vi "ServerPolicy.vi"(3 "xml content":string="<?xml version=\"1.0\" encoding=\"utf-8\"?><opcua_server><name>Faraday Cup Control System</name><port>4845</port><policy>none</policy><serverCertification></serverCertification><trustedClientCertifications>  <certification></certification></trustedClientCertifications><structure>    <folder name=\"System\">        <item name=\"Server URL\" ,access=\"read/write\" datatype=\"string\" initialValue=\"\" description=\"Server URL.\"></item>    </folder>    <folder name=\"Motion\">        <folder name=\"Contorl\">            <item name=\"Power Enable\" access=\"read/write\" datatype=\"boolean\" initialValue=\"FALSE\" description=\"Enable the motion power.\"></item>            <item name=\"Start Move\" access=\"read/write\" datatype=\"boolean\" initialValue=\"FALSE\" description=\"Start to move.\"></item>            <item name=\"Stop Move\" access=\"read/write\" datatype=\"boolean\" initialValue=\"FALSE\" description=\"Stop the movement.\"></item>            <item name=\"Find Home\" access=\"read/write\" datatype=\"boolean\" initialValue=\"FALSE\" description=\"Start to find home.\"></item>        </folder>        <folder name=\"Status\">            <item name=\"FWD Limit\" access=\"read\" datatype=\"boolean\" initialValue=\"FALSE\" description=\"Show the status of fwd limit.\"></item>            <item name=\"REV Limit\" access=\"read\" datatype=\"boolean\" initialValue=\"FALSE\" description=\"Show the status of rev limit.\"></item>            <item name=\"STO\" access=\"read\" datatype=\"boolean\" initialValue=\"FALSE\" description=\"Show the status of STO.\"></item>            <item name=\"Move Complete\" access=\"read\" datatype=\"boolean\" initialValue=\"FALSE\" description=\"Show the status of movement.\"></item>            <item name=\"Find Home Complete\" access=\"read\" datatype=\"boolean\" initialValue=\"FALSE\" description=\"show the status of finding home.\"></item>            <item name=\"E Ruler\" access=\"read\" datatype=\"double\" initialValue=\"0\" description=\"Show the Eruler position.\"></item>        </folder>        <folder name=\"Last Error\">            <item name=\"acknowledge\" access=\"read/write\" datatype=\"boolean\" initialValue=\"FALSE\" description=\"Acknowledge last error.\"></item>            <item name=\"code\" access=\"read\" datatype=\"int32\" initialValue=\"0\" description=\"Show the code of last error.\"></item>            <item name=\"info\" access=\"read\" datatype=\"int32\" initialValue=\"0\" description=\"Show the info of last error.\"></item>        </folder>    </folder>    <folder name=\"DAQ\">        <item name=\"Measurement Range\" access=\"read/write\" datatype=\"int16\" initialValue=\"100\" description=\"Measurement range.\"></item>        <item name=\"Intensity\" access=\"read\" datatype=\"double\" initialValue=\"100\" description=\"Intensity Value.\"></item>        <item name=\"Save file?\" access=\"read/write\" datatype=\"boolean\" initialValue=\"FALSE\" description=\"Enable saving file.\"></item>        <item name=\"File Path\" access=\"read/write\" datatype=\"string\" initialValue=\"\" description=\"Local path of saved file.\"></item>    </folder></structure></opcua_server>") -> (0 "security policy":T1, 1 "xml content(dup)":string)   [LabVIEW 2013, in "OPCUA XML.lvlib"]
uses:
  OPCUA XML.lvlib
panel:
  out "result string":string
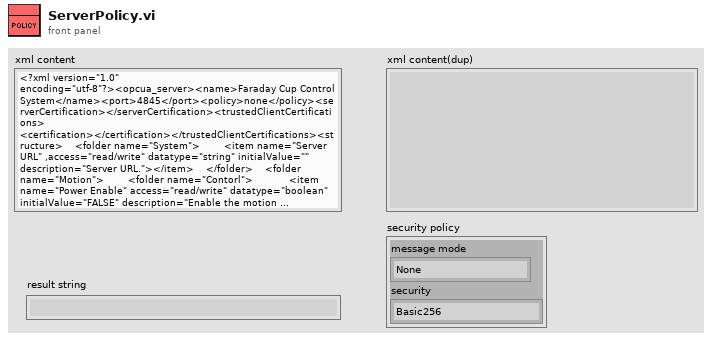
[diagram p1: front panel]
types:
  T1 = cluster{"message mode":enum16{"None", "Sign", "Sign and Encrypt"}, "security":enum16{"Basic256", "Basic128Rsa15"}}
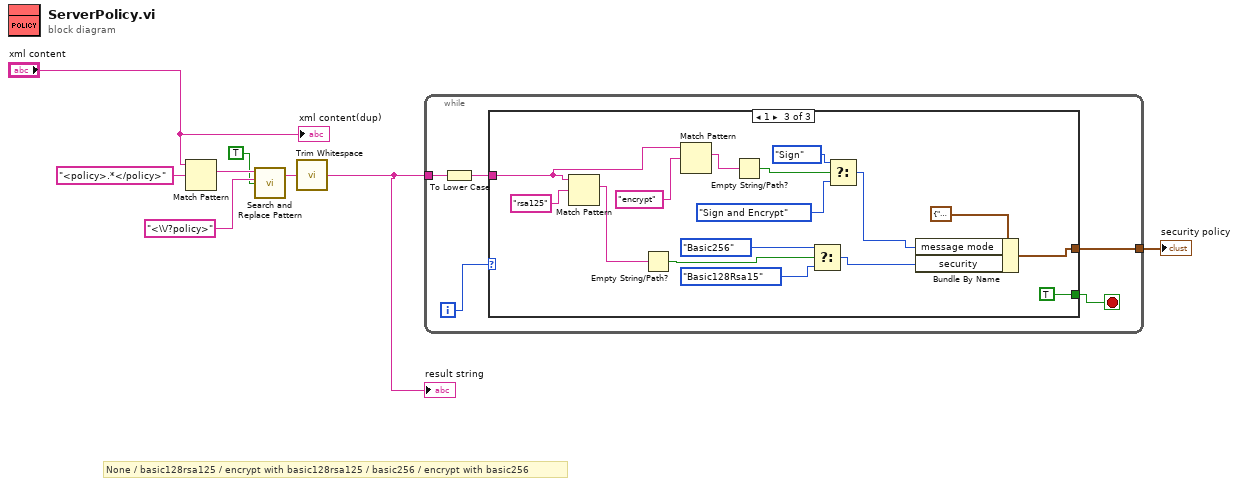
[diagram p0: block diagram]
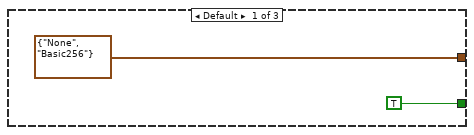
[diagram p2: hidden frame]
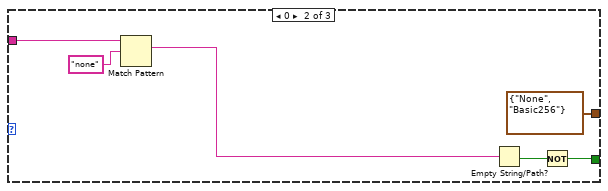
[diagram p3: hidden frame]
diagram:
  # "None / basic128rsa125 / encrypt with basic128rsa125 / basic256 / encrypt with basic256"
  n1 = Match Pattern(string="xml content", regular expression="<policy>.*</policy>") -> (match substring=w7:string)  [unwired: 1 in, 3 out]
  n2 = call <vilib>:"Search and Replace Pattern.vi"("string"=w7, "regular expression (\"\")"="<\\/?policy>" ("regular expression"), "replace all? (F)"=TRUE) -> ("result string"=w5:string)  [unwired: 2 in, 1 out]
  n3 = call <vilib>:"Trim Whitespace.vi"("string"=w5) -> ("trimmed string"=w1:string)  [unwired: 1 in]
  "result string" <- w1
  n4 = while {
    tunnel: w1 -> [w13]
    tunnel: [w10] -> w2
    i -> [w11]
    stop <- w9 stop-if-true
    n5 = To Lower Case(string=w13) -> (all lower case string=w12:string)
    n6 = case shown="1" w11 {
      tunnel: w12 -> [_ w21 w32]
      tunnel: [TRUE w19 TRUE] -> w9
      tunnel: [T1 {"message mode"=enum."None", "security"=enum."Basic256"} ("security policy") T1 {"message mode"=enum."None", "security"=enum."Basic256"} ("security policy") w23] -> w10
      frame Default {
      }
      frame 0 {
        n7 = Match Pattern(string=w21, regular expression="none") -> (match substring=w17:string)  [unwired: 1 in, 3 out]
        n8 = Empty String/Path?(string/path=w17) -> (empty?=w18:bool)
        n9 = Not(x=w18) -> (.not. x?=w19:bool)
      }
      frame 1 {
        n10 = Match Pattern(string=w32, regular expression="rsa125") -> (match substring=w36:string)  [unwired: 1 in, 3 out]
        n11 = Empty String/Path?(string/path=w36) -> (empty?=w33:bool)
        n12 = Match Pattern(string=w32, regular expression="encrypt") -> (match substring=w30:string)  [unwired: 1 in, 3 out]
        n13 = Empty String/Path?(string/path=w30) -> (empty?=w27:bool)
        n14 = Select(t=enum16{"Basic256", "Basic128Rsa15"}."Basic256" ("security"), s=w33, f=enum16{"Basic256", "Basic128Rsa15"}."Basic128Rsa15" ("security")) -> (s? t:f=w24:enum16{"Basic256", "Basic128Rsa15"})
        n15 = Select(t=enum16{"None", "Sign", "Sign and Encrypt"}."Sign" ("message mode"), s=w27, f=enum16{"None", "Sign", "Sign and Encrypt"}."Sign and Encrypt" ("message mode")) -> (s? t:f=w25:enum16{"None", "Sign", "Sign and Encrypt"})
        n16 = Bundle By Name(cluster=T1 {"message mode"=enum."None", "security"=enum."Basic256"} ("security policy"), "message mode"=w25, "security"=w24) -> (w23:T1)
      }
    }
  }
  "security policy" <- w2
  "xml content(dup)" <- "xml content"
